vi "Muxed_Stram_withDC.vi"() -> ()   [LabVIEW 2014]
uses:
  <vilib>/FPGAPlugInAG/PXI-7852R/niLvFpga_Open_PXI-7852R.vi
  <vilib>/rvi/interface/common/dynamic/niFpgaDynamicAddResources.vi
  <vilib>/Utility/error.llb/Error Cluster From Error Code.vi
  <vilib>/rvi/errors/niLvFpgaAdjustHostInterfaceError.vi
  <vilib>/Utility/file.llb/Write To Spreadsheet File (I64).vi
  <vilib>/measure/maspectr.llb/FFT Power Spectrum and PSD for 1 Chan.vi
  <vilib>/FPGAPlugInAG/Dynamic/niLvFpga_Close_Dynamic.vi
  <vilib>/rvi/interface/nirviOpenFPGA/nirviOpenFPGA.xnode
  FPGA Bitfiles/MilitaruDAQ_FPGATarget_MuxedAcquisition_glcrRcw8lng.lvbitx
  <vilib>/rvi/interface/nirviMethod/nirviMethod.xnode
  <vilib>/rvi/interface/nirviReadWriteControl/nirviReadWriteControl.xnode
  <vilib>/rvi/interface/nirviCloseFPGA/nirviCloseFPGA.xnode
  <vilib>/FPGAPlugInAG/Dynamic/niLvFpga_ReadFifo_Dynamic.vi
  <vilib>/rvi/errors/niLvFpgaMergeErrorWithErrorCode.vi
  NiFpgaLv.dll
  <vilib>/rvi/interface/Simulation/niFpgaSimulationCallBeginRW.vi
  <vilib>/measure/NI_MAPro.lvlib
panel:
  out "DC":i16[](array[numeric])
  out "DC-sample [Hz]":dbl
  in  "Number of Elements":u32
  out "Position":waveform(i16)(graph) caption="Dynamic Data Type"
  in  "dB On (F)":bool
  in  "averaging parameters":T1={"averaging mode"=enum."No averaging", "weighting mode"=enum."Exponential", "number of averages"=10} {"number of averages" min=1}
  out "PSD":cluster{"f0":dbl, "df":dbl, "magnitude":dbl[]}(graph) caption="Dynamic Data Type"
  in  "file path (dialog if empty)":path
  in  "append to file? (new file:F)":bool
  in  "Sampling(Ticks)":u32
  out "Sampling Frequency\n(kHz)":dbl
  out "Acquisition Timeout":bool
  out "FIFO timeout":bool
  in  "Acquisition-Channel":i16
  in  "DC sampling":u32
  in  "DC Elements":u32
  out "DC elements remaining":u32
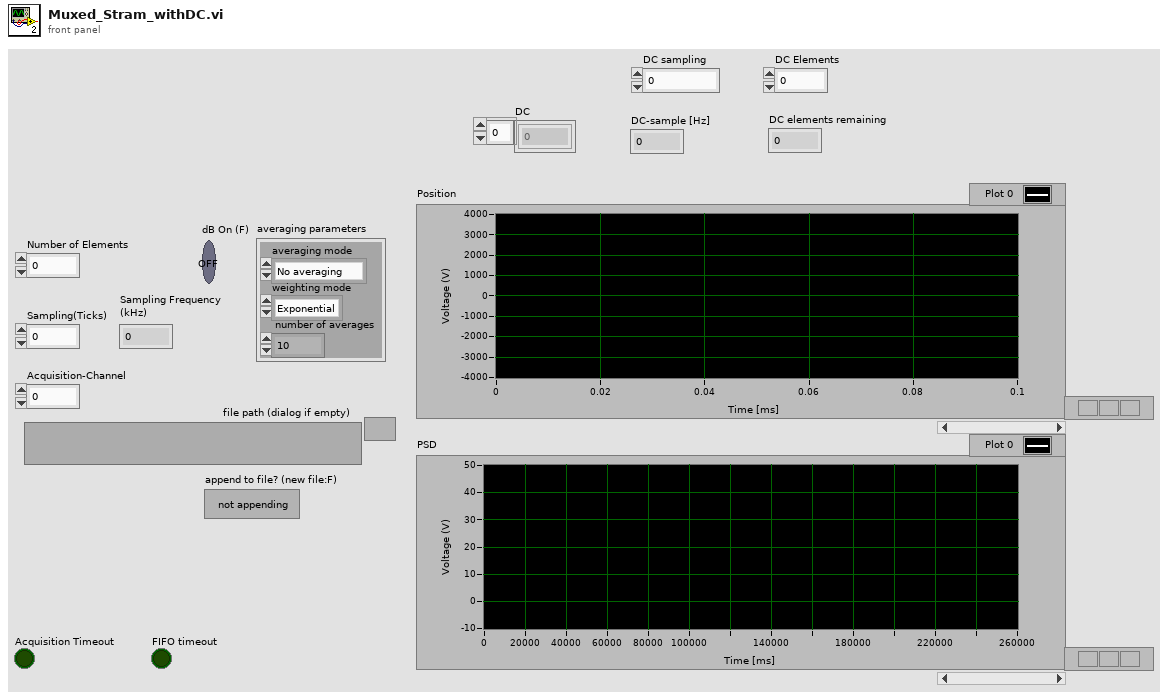
[diagram p1: front panel]
types:
  T1 = cluster{"averaging mode":enum16{"No averaging", "Vector averaging", "RMS averaging", "Peak hold"}, "weighting mode":enum16{"Linear", "Exponential"}, "number of averages":u32}
  T2 = enum16{"open", "replace", "create", "open or create", "replace or create", "replace or create with confirmation"}
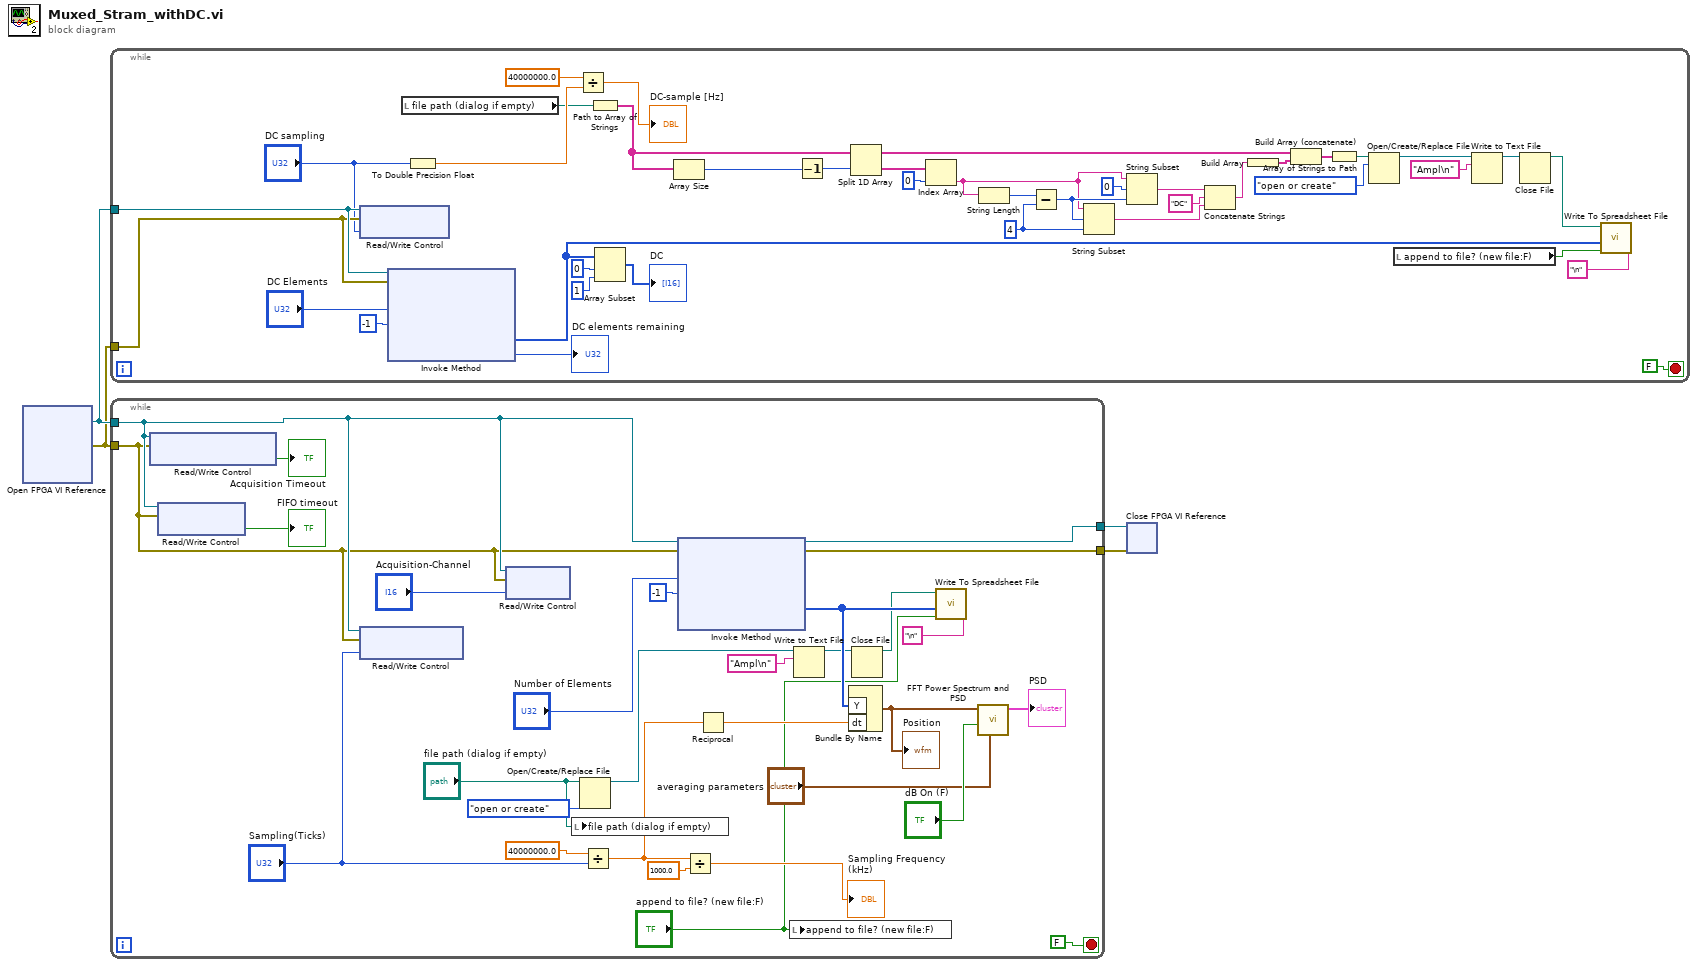
[diagram p0: block diagram]
diagram:
  n1 = xnode "Open FPGA VI Reference"() -> ("FPGA VI Reference Out"=w2:refnum<k20>, "error out"=w1:errorcluster)  [unwired: 2 in]
  n2 = while {
    tunnel: w2 -> [w38]
    tunnel: w1 -> [w37]
    stop <- FALSE stop-if-true
    w25 = 4 ("y")
    n3 = xnode "Read/Write Control"("FPGA VI Reference In"=w38, "error in"=w37, "DC-Sampling"="DC sampling") -> ()  [unwired: 2 out]
    n4 = xnode "Invoke Method"("FPGA VI Reference In"=w38, "error in"=w37, "Number of Elements"="DC Elements", "Timeout (ms)"=-1) -> ("Data"=w6:i16[], "Elements Remaining"=→"DC elements remaining":u32)  [unwired: 2 out]
    n5 = local read "file path (dialog if empty)"() -> (w32:path)
    n6 = To Double Precision Float(number="DC sampling") -> (double precision float=w42:dbl)
    n7 = Divide(x=40000000.0, y=w42) -> (x/y=→"DC-sample [Hz]":dbl)
    n8 = Path to Array of Strings(0:w32) -> (2:w31:string[])  [unwired: 1 out]
    n9 = Array Subset(array=w6, index=0, length=1) -> (→"DC":i16[])
    n10 = Array Size(array=w31) -> (size(s)=w30:i32)
    n11 = Decrement(x=w30) -> (x-1=w29:i32)
    n12 = Split 1D Array(array=w31, index=w29) -> (first subarray=w16:string[], second subarray=w27:string[])
    n13 = Index Array(array=w27, index=0) -> (element=w22:string)
    n14 = String Length(string=w22) -> (length=w26:i32)
    n15 = Subtract(x=w26, y=w25) -> (x-y=w23:i32)
    n16 = String Subset(string=w22, offset (0)=w23, length (rest)=w25) -> (substring=w20:string)
    n17 = String Subset(string=w22, offset (0)=0, length (rest)=w23) -> (substring=w21:string)
    n18 = Concatenate Strings(w21, "DC" ("string"), w20) -> (w18:string)
    n19 = Build Array(w18) -> (w17:string[])
    n20 = Build Array (concatenate)(w16, w17) -> (w15:string[])
    n21 = Array of Strings to Path(0:w15) -> (2:w8:path)  [unwired: 1 in]
    n22 = Open/Create/Replace File(file path (use dialog)=w8, operation (0:open)=T2."open or create") -> (refnum out=w11:refnum<file>)  [unwired: 4 in, 2 out]
    n23 = local read "append to file? (new file:F)"() -> (w7:bool)
    n24 = Write to Text File(file (use dialog)=w11, text="Ampl\n") -> (refnum out=w10:refnum<file>)  [unwired: 2 in, 2 out]
    n25 = Close File(refnum=w10) -> (path=w5:path)  [unwired: 1 in, 1 out]
    n26 = call-poly <vilib>:"Write To Spreadsheet File.vi"("delimiter (\\t)"="\n" ("delimiter (\\t)"), "append to file? (new file:F)"=w7, "1D data"=w6, "file path (dialog if empty)"=w5) -> ()  [unwired: 4 in, 1 out]
  }
  n27 = while {
    tunnel: w2 -> [w53]
    tunnel: w1 -> [w52]
    tunnel: [w66] -> w3
    tunnel: [w65] -> w4
    stop <- FALSE stop-if-true
    n28 = xnode "Read/Write Control"("FPGA VI Reference In"=w53, "error in"=w52) -> ("Acquisition Timeout"=→"Acquisition Timeout":bool)  [unwired: 2 out]
    n29 = xnode "Read/Write Control"("FPGA VI Reference In"=w53, "error in"=w52) -> ("FIFO timeout"=→"FIFO timeout":bool)  [unwired: 2 out]
    n30 = xnode "Read/Write Control"("FPGA VI Reference In"=w53, "error in"=w52, "Sampling(Ticks)"="Sampling(Ticks)") -> ()  [unwired: 2 out]
    n31 = xnode "Read/Write Control"("FPGA VI Reference In"=w53, "error in"=w52, "Numeric"="Acquisition-Channel") -> ()  [unwired: 2 out]
    n32 = local write "file path (dialog if empty)"("file path (dialog if empty)") -> ()
    n33 = Open/Create/Replace File(file path (use dialog)="file path (dialog if empty)", operation (0:open)=T2."open or create") -> (refnum out=w61:refnum<file>)  [unwired: 4 in, 2 out]
    n34 = Divide(x=40000000.0, y="Sampling(Ticks)") -> (x/y=w49:dbl)
    n35 = xnode "Invoke Method"("FPGA VI Reference In"=w53, "error in"=w52, "Number of Elements"="Number of Elements", "Timeout (ms)"=-1) -> ("FPGA VI Reference Out"=w66:refnum<k20>, "error out"=w65:errorcluster, "Data"=w64:i16[])  [unwired: 1 out]
    n36 = Divide(x=w49, y=1000.0) -> (x/y=→"Sampling Frequency\n(kHz)":dbl)
    n37 = Reciprocal(x=w49) -> (1/x=w56:dbl)
    n38 = local write "append to file? (new file:F)"("append to file? (new file:F)") -> ()
    n39 = Write to Text File(file (use dialog)=w61, text="Ampl\n") -> (refnum out=w60:refnum<file>)  [unwired: 2 in, 2 out]
    n40 = Bundle By Name ("Build Waveform")("Y"=w64, "dt"=w56) -> (w70:waveform(i16))  [unwired: 1 in]
    "Position" <- w70
    n41 = Close File(refnum=w60) -> (path=w59:path)  [unwired: 1 in, 1 out]
    n42 = call-poly <vilib>:"Write To Spreadsheet File.vi"("delimiter (\\t)"="\n" ("delimiter (\\t)"), "append to file? (new file:F)"="append to file? (new file:F)", "1D data"=w64, "file path (dialog if empty)"=w59) -> ()  [unwired: 4 in, 1 out]
    n43 = call-poly <vilib>:"FFT Power Spectrum and PSD.vi"("averaging parameters"="averaging parameters", "dB On (F)"="dB On (F)", "time signal"=w70) -> ("Power Spectrum / PSD"=→"PSD":cluster{"f0":dbl, "df":dbl, "magnitude":dbl[]})  [unwired: 5 in, 3 out]
  }
  n44 = xnode "Close FPGA VI Reference"("FPGA VI Reference In"=w3, "error in"=w4) -> ()  [unwired: 1 out]
